vi "HandleItemActivation.vi"(8 "error in (no error)":errorcluster, 11 "GettingStartedWindow.lvlib:RingItemVINoParams.lvclass":refnum<class "RingItemVINoParams.lvclass">) -> (0 "error out":errorcluster, 3 "GettingStartedWindow.lvlib:RingItemVINoParams.lvclass 2":refnum<class "RingItemVINoParams.lvclass">)   [LabVIEW 2009, in "NavScreen.lvlib" / "RingItemVINoParams.lvclass"]
uses:
  RingItemVINoParams.lvclass
  RingItemVINoParams.lvclass/RingItemVINoParams.ctl
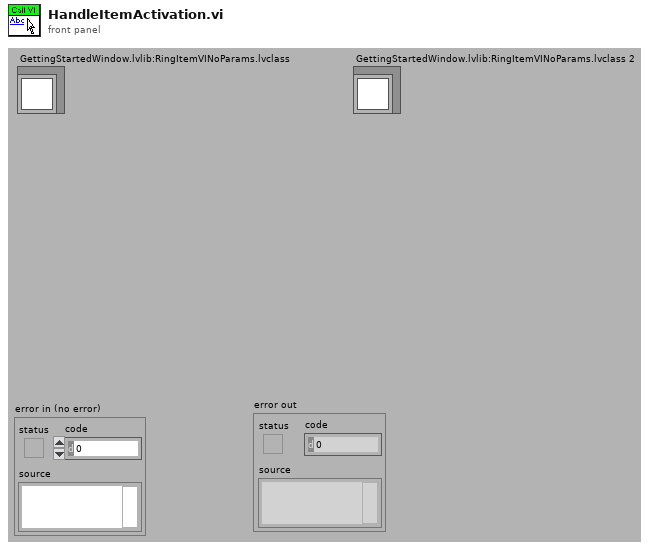
[diagram p1: front panel]
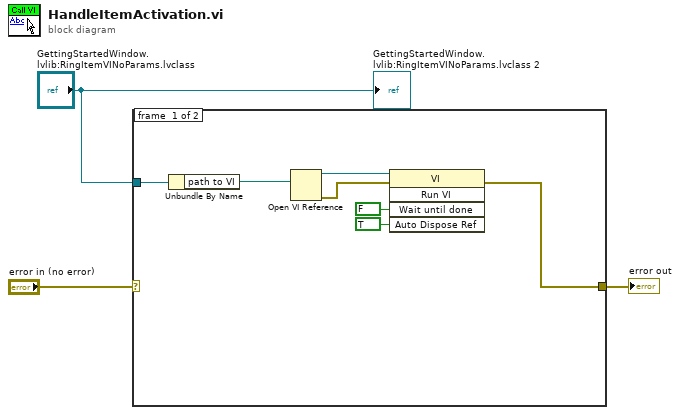
[diagram p0: block diagram]
diagram:
  n1 = case shown="No Error" "error in (no error)" {
    selector: "error in (no error)" -> [_ w11]
    tunnel: [w6 w11] -> w2
    tunnel: "GettingStartedWindow.lvlib:RingItemVINoParams.lvclass" -> [w5 _]
    frame #0 {
      n2 = Unbundle By Name(w5) -> ("path to VI"=w4:path)
      n3 = Open VI Reference(vi path=w4) -> (vi reference=w9:refnum<vi>, error out=w10:errorcluster)  [unwired: 5 in]
      n4 = invoke class="VI" method="Run VI"(reference=w9, error in=w10, "Wait until done"=FALSE ("Wait Until Done"), "Auto Dispose Ref"=TRUE ("Auto Dispose Reference")) -> (error out=w6:errorcluster)  [unwired: 1 in, 4 out]
    }
    frame #1 {
    }
  }
  "error out" <- w2
  "GettingStartedWindow.lvlib:RingItemVINoParams.lvclass 2" <- "GettingStartedWindow.lvlib:RingItemVINoParams.lvclass"
